vi "LVJSON Create.vi"(9 "Variant (Void=Default Type)":variant, 10 "Type":T1, 11 "Key":string) -> (3 "Element out":T2)   [LabVIEW 2019, in "labview_json.lvlib"]
uses:
  labview_json.lvlib
  Element.ctl
  Element Type.ctl
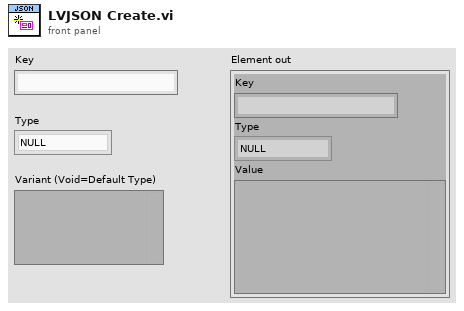
[diagram p1: front panel]
types:
  T1 = typedef "labview_json.lvlib/Element Type.ctl" = enum8{"NULL", "OBJECT", "ARRAY", "BOOL", "INT", "UINT", "FLOAT", "STRING"}
  T2 = typedef "labview_json.lvlib/Element.ctl" = cluster{"Key":string, "Type":T1, "Value":variant}
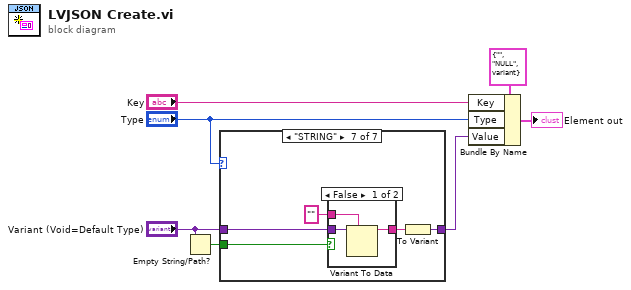
[diagram p0: block diagram]
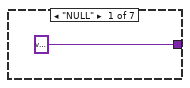
[diagram p2: hidden frame]
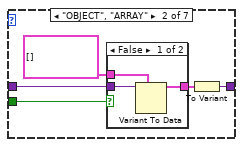
[diagram p3: hidden frame]
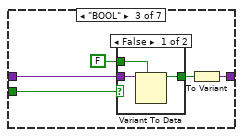
[diagram p5: hidden frame]
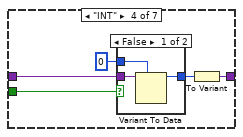
[diagram p7: hidden frame]
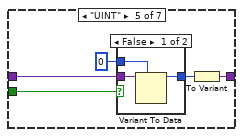
[diagram p9: hidden frame]
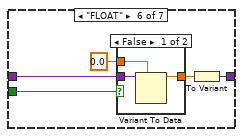
[diagram p11: hidden frame]
diagram:
  n1 = Empty String/Path?(string/path="Variant (Void=Default Type)") -> (empty?=w1:bool)
  n2 = case shown="\"STRING\"" "Type" {
    tunnel: "Variant (Void=Default Type)" -> [_ w13 w22 w31 w40 w49 w58]
    tunnel: [variant ("Variant") w10 w20 w29 w38 w47 w56] -> w3
    tunnel: w1 -> [_ w9 w18 w28 w37 w46 w55]
    frame "NULL" {
    }
    frame "OBJECT", "ARRAY" {
      n3 = case shown="False" w9 {
        tunnel: w13 -> [w16 _]
        tunnel: T2[] [] -> [w15 w17]
        tunnel: [w14 w17] -> w11
        frame False {
          n4 = Variant To Data(type=w15, Variant=w16) -> (data=w14:T2[])  [unwired: 1 in, 1 out]
        }
        frame True {
        }
      }
      n5 = To Variant(anything=w11) -> (Variant=w10:variant)
    }
    frame "BOOL" {
      n6 = case shown="False" w18 {
        tunnel: w22 -> [w25 _]
        tunnel: [w24 w26] -> w21
        tunnel: FALSE -> [w23 w26]
        frame False {
          n7 = Variant To Data(type=w23, Variant=w25) -> (data=w24:bool)  [unwired: 1 in, 1 out]
        }
        frame True {
        }
      }
      n8 = To Variant(anything=w21) -> (Variant=w20:variant)
    }
    frame "INT" {
      n9 = case shown="False" w28 {
        tunnel: w31 -> [w34 _]
        tunnel: [w33 w35] -> w30
        tunnel: i64 0 -> [w32 w35]
        frame False {
          n10 = Variant To Data(type=w32, Variant=w34) -> (data=w33:i64)  [unwired: 1 in, 1 out]
        }
        frame True {
        }
      }
      n11 = To Variant(anything=w30) -> (Variant=w29:variant)
    }
    frame "UINT" {
      n12 = case shown="False" w37 {
        tunnel: w40 -> [w43 _]
        tunnel: [w42 w44] -> w39
        tunnel: u64 0 -> [w41 w44]
        frame False {
          n13 = Variant To Data(type=w41, Variant=w43) -> (data=w42:u64)  [unwired: 1 in, 1 out]
        }
        frame True {
        }
      }
      n14 = To Variant(anything=w39) -> (Variant=w38:variant)
    }
    frame "FLOAT" {
      n15 = case shown="False" w46 {
        tunnel: w49 -> [w52 _]
        tunnel: [w51 w53] -> w48
        tunnel: 0.0 -> [w50 w53]
        frame False {
          n16 = Variant To Data(type=w50, Variant=w52) -> (data=w51:dbl)  [unwired: 1 in, 1 out]
        }
        frame True {
        }
      }
      n17 = To Variant(anything=w48) -> (Variant=w47:variant)
    }
    frame "STRING" {
      n18 = case shown="False" w55 {
        tunnel: w58 -> [w61 _]
        tunnel: [w60 w62] -> w57
        tunnel: "" -> [w59 w62]
        frame False {
          n19 = Variant To Data(type=w59, Variant=w61) -> (data=w60:string)  [unwired: 1 in, 1 out]
        }
        frame True {
        }
      }
      n20 = To Variant(anything=w57) -> (Variant=w56:variant)
    }
  }
  n21 = Bundle By Name(cluster=T2 {"Key"="", "Type"=enum."NULL", "Value"=variant} ("Element out"), "Key"="Key", "Type"="Type", "Value"=w3) -> (→"Element out":T2)
